vi "Write Config.vi"(8 "error in (no error)":errorcluster, 10 "Config":variant, 11 "ProjectLoader in":refnum<class "ProjectLoader.lvclass">) -> (0 "error out":errorcluster, 3 "ProjectLoader out":refnum<class "ProjectLoader.lvclass">)   [LabVIEW 2015, in "ProjectLoader.lvclass"]
uses:
  ProjectLoader.lvclass
  ProjectLoader.lvclass/ProjectLoader.ctl
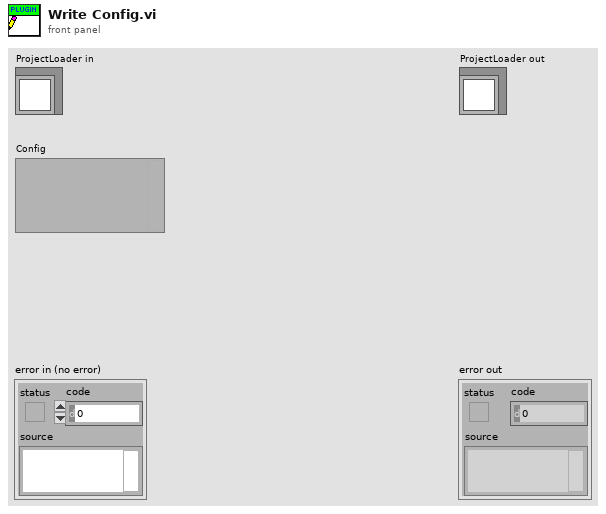
[diagram p1: front panel]
types:
  T1 = cluster{"Enable":bool, "Auto Load":bool, "Project File":path}
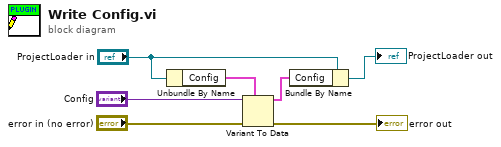
[diagram p0: block diagram]
diagram:
  n1 = Unbundle By Name("ProjectLoader in") -> ("Config"=w7:T1)
  n2 = Variant To Data(error in="error in (no error)", type=w7, Variant="Config") -> (data=w3:T1, error out=→"error out":errorcluster)
  n3 = Bundle By Name(cluster="ProjectLoader in", "Config"=w3) -> (→"ProjectLoader out":refnum<class "ProjectLoader.lvclass">)
